vi "Write_Growth_DBorig.vi"(0 "Growth Name":string, 1 "Notes":string, 2 "Log File":path, 3 "Growth Sequence File":path, 4 "Operator Name":string) -> (5 "Error":bool)   [LabVIEW 2011]
uses:
  low_level_proc/globals.vi
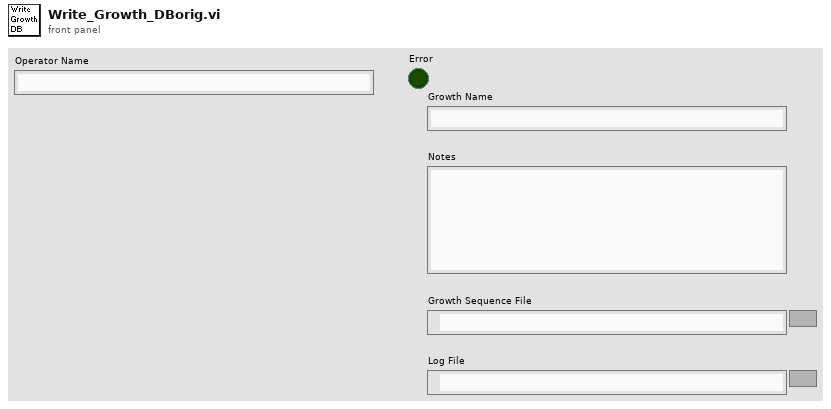
[diagram p1: front panel]
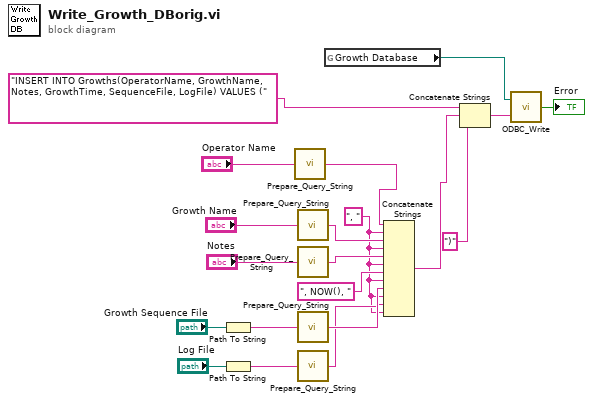
[diagram p0: block diagram]
diagram:
  w1 = ", " ("string")
  n1 = Path To String(path="Growth Sequence File") -> (string=w12:string)
  n2 = Path To String(path="Log File") -> (string=w10:string)
  n3 = call "Prepare_Query_String.vi"("Input String"="Operator Name") -> ("Output String"=w9:string)
  n4 = call "Prepare_Query_String.vi"("Input String"="Growth Name") -> ("Output String"=w8:string)
  n5 = call "Prepare_Query_String.vi"("Input String"="Notes") -> ("Output String"=w7:string)
  n6 = call "Prepare_Query_String.vi"("Input String"=w12) -> ("Output String"=w5:string)
  n7 = call "Prepare_Query_String.vi"("Input String"=w10) -> ("Output String"=w4:string)
  n8 = global read "globals.vi" "Growth Database"() -> (w16:path)
  n9 = Concatenate Strings(w9, w1, w8, w1, w7, w1, ", NOW(), " ("string"), w1, w5, w1, w4, w1) -> (w3:string)
  n10 = Concatenate Strings("INSERT INTO Growths(OperatorName, GrowthName, Notes, GrowthTime, SequenceFile, LogFile) VALUES (" ("string"), w3, ")" ("string")) -> (w19:string)
  n11 = call "ODBC_Write.vi"("Query"=w19, "Database File"=w16) -> ("Error"=→"Error":bool)
